vi "OAT_Display_Freq-RPM Map_Easy.vi"(4 "window info":T1={"window type"=3, "window length"=2048} {"window type" items=["None"=0, "Hanning"=1, "Hamming"=2, "Blackman-Harris"=3, "Exact Blackman"=4, "Blackman"=5, "Flat Top"=6, "4 Term B-Harris"=7, "7 Term B-Harris"=8, "Low Sidelobe"=9, "Gaussian"=62]; "window length" min=0}, 8 "pulse/revolution (1)":dbl=1.0 format="%.2f", 9 "analog tach signal":waveform(dbl)={"t0"=timestamp(0 s since 1904-01-01), "dt"=0.0, "Y"=[]}, 11 "scaled signal [EU]":waveform(dbl)={"t0"=timestamp(0 s since 1904-01-01), "dt"=0.0, "Y"=[]}) -> (1 "Selected Order":dbl=1.0 format="%.1f", 3 "Campbell Diagram":picture)   [LabVIEW 2017]
uses:
  <vilib>/addons/Sound and Vibration/Order Analysis/Ref Gabor Order Tracking/window information.ctl
  <vilib>/addons/Sound and Vibration/Order Analysis/Gabor Order Tracking/SoundVib_Gabor.lvlib
  <vilib>/addons/Sound and Vibration/Order Analysis/Tach Process/SoundVib_TachProcess.lvlib
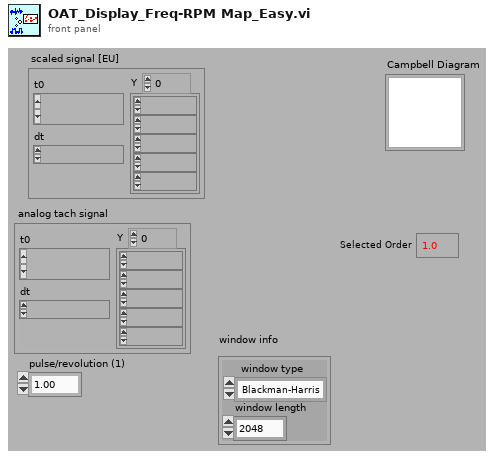
[diagram p1: front panel]
types:
  T1 = typedef "SoundVib_Gabor.lvlib/window information.ctl" = cluster{"window type":u32, "window length":i32}
  T2 = typedef "SoundVib_Gabor.lvlib/GT RefNum.ctl" = refnum<k1>
  T3 = typedef "SoundVib_TachProcess.lvlib/speed profile.ctl" = cluster{"time [s]":dbl[], "speed [RPM]":dbl[]}
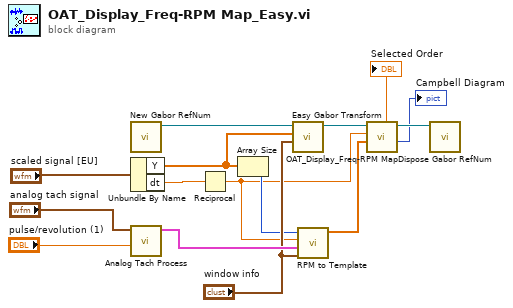
[diagram p0: block diagram]
diagram:
  n1 = call <vilib>:"New Gabor RefNum.vi"() -> ("RefNum"=w15:T2)  [unwired: 9 in, 1 out]
  n2 = Unbundle By Name("scaled signal [EU]") -> ("Y"=w10:dbl[], "dt"=w13:dbl)
  n3 = call <vilib>:"Analog Tach Process.vi"("pulse/revolution (1)"="pulse/revolution (1)", "analog tach signal"="analog tach signal") -> ("speed profile"=w14:T3)  [unwired: 7 in, 2 out]
  n4 = Reciprocal(x=w13) -> (1/x=w8:dbl)
  n5 = Array Size(array=w10) -> (size(s)=w11:i32)
  n6 = call <vilib>:"Easy Gabor Transform.vi"("window info"="window info", "x[n]"=w10, "RefNum in"=w15) -> ("RefNum out"=w9:T2)  [unwired: 4 in, 4 out]
  n7 = call <vilib>:"RPM to Template.vi"("window info"="window info", "speed profile"=w14, "sampling frequency [Hz]"=w8, "signal length"=w11) -> ("Gabor template"=w7:dbl[])  [unwired: 6 in, 1 out]
  n8 = call <vilib>:"OAT_Display_Freq-RPM Map.vi"("Gabor Template"=w7, "sampling frequency (Hz)"=w8, "Gabor RefNum"=w9) -> ("Diagram"=→"Campbell Diagram":picture, "Gabor RefNum Out"=w6:T2, "Order"=→"Selected Order":dbl)  [unwired: 4 in, 2 out]
  n9 = call <vilib>:"Dispose Gabor RefNum.vi"("RefNum in"=w6) -> ()  [unwired: 7 in, 1 out]
